vi "ReadFITS2SGL.vi"(8 "Error In":errorcluster, 11 "Path":path) -> (0 "error out":errorcluster, 1 "Tableau2DSGL":sgl[][][](array[numeric]), 2 "Tableau2DSGL":sgl[][](array[numeric]), 3 "Tableau_1D_SGL":sgl[](array[numeric]))   [LabVIEW 2020]
doc: "Relecture de fichier FITS. \nLes données sont relues au format SGL. Il y a un problème avec la lecture des données en U16. On les relit comme des entiers signés et j'ajoute la valeur 32768."
panel:
  out "Header":T1={"Naxis"=0, "Naxis1"=0, "Naxis2"=0, "Naxis3"=0, "DataType"=32, "Bscale"=0.0, "Bzero"=0.0} {"DataType" items=["U8"=8, "I16"=16, "I32"=32, "SGL (float)"=-32, "DBL"=-64]}
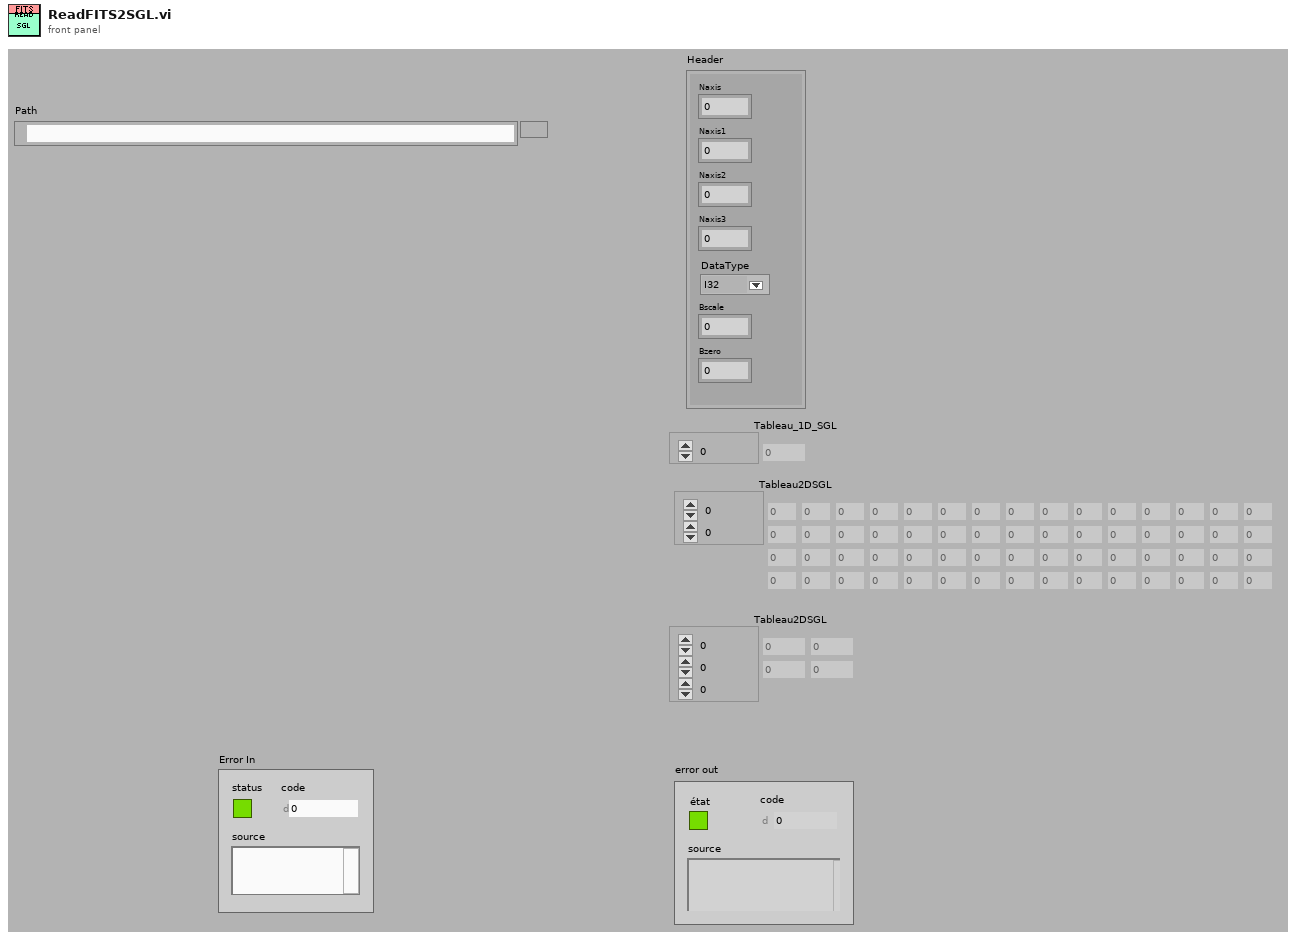
[diagram p1: front panel]
types:
  T1 = cluster{"Naxis":i32, "Naxis1":i32, "Naxis2":i32, "Naxis3":i32, "DataType":i32, "Bscale":dbl, "Bzero":dbl}
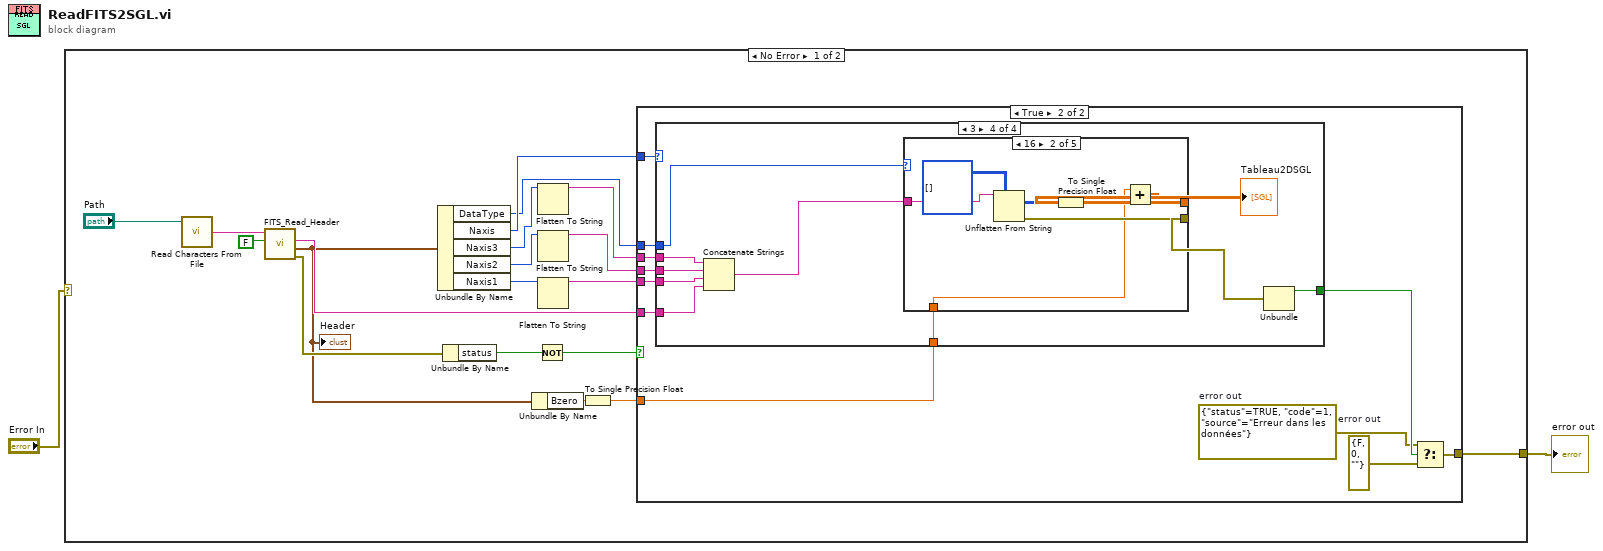
[diagram p0: block diagram]
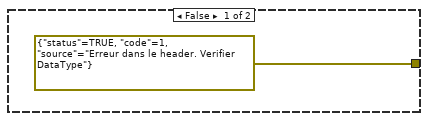
[diagram p2: hidden frame]
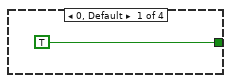
[diagram p3: hidden frame]
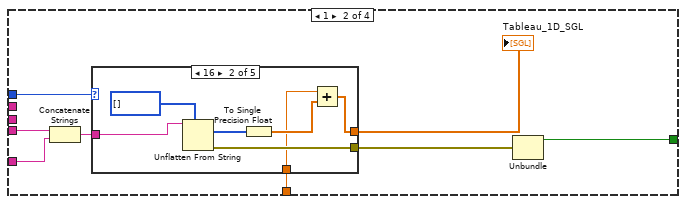
[diagram p4: hidden frame]
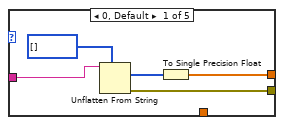
[diagram p5: hidden frame]
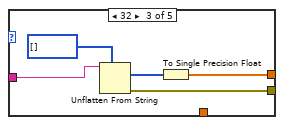
[diagram p6: hidden frame]
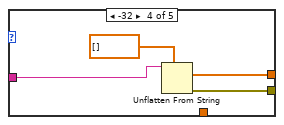
[diagram p7: hidden frame]
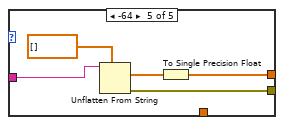
[diagram p8: hidden frame]
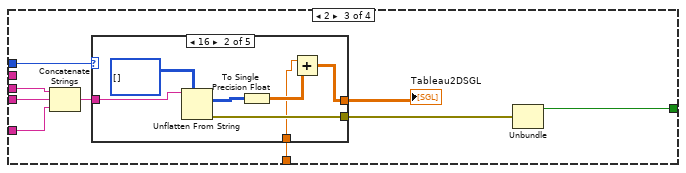
[diagram p9: hidden frame]
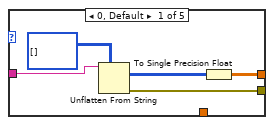
[diagram p10: hidden frame]
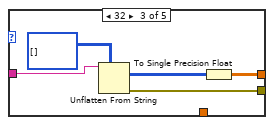
[diagram p11: hidden frame]
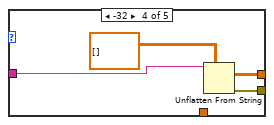
[diagram p12: hidden frame]
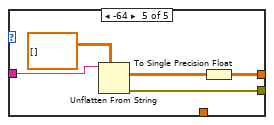
[diagram p13: hidden frame]
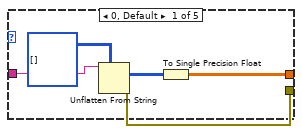
[diagram p14: hidden frame]
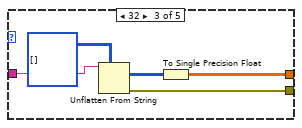
[diagram p15: hidden frame]
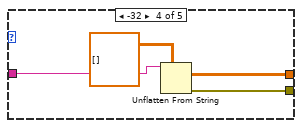
[diagram p16: hidden frame]
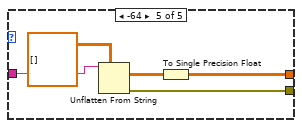
[diagram p17: hidden frame]
diagram:
  n1 = case shown="No Error" "Error In" {
    selector: "Error In" -> [_ w140]
    tunnel: [w6 w140] -> w2
    frame No Error {
      n2 = call <vilib>:"Read Characters From File.vi"("file path (dialog if empty)"="Path") -> ("character string"=w9:string)  [unwired: 5 in, 3 out]
      n3 = call "FITS_Read_Header.vi"("Load ?"=FALSE, "FITS in"=w9) -> ("error out"=w20:errorcluster, "Header"=w5:T1, "FITS data"=w15:string)  [unwired: 2 in, 1 out]
      "Header" <- w5
      n4 = Unbundle By Name(w5) -> ("DataType"=w7:i32, "Naxis"=w18:i32, "Naxis3"=w12:i32, "Naxis2"=w13:i32, "Naxis1"=w14:i32)
      n5 = Unbundle By Name(w20) -> ("status"=w19:bool)
      n6 = Unbundle By Name(w5) -> ("Bzero"=w4:dbl)
      n7 = Not(x=w19) -> (.not. x?=w10:bool)
      n8 = Flatten To String(anything=w12) -> (data string=w11:string)  [unwired: 3 in, 2 out]
      n9 = Flatten To String(anything=w13) -> (data string=w16:string)  [unwired: 3 in, 2 out]
      n10 = Flatten To String(anything=w14) -> (data string=w17:string)  [unwired: 3 in, 2 out]
      n11 = To Single Precision Float(number=w4) -> (single precision float=w3:sgl)
      n12 = case shown="True" w10 {
        tunnel: w17 -> [_ w32]
        tunnel: w18 -> [_ w33]
        tunnel: [errorcluster {"status"=TRUE, "code"=1, "source"="Erreur dans le header. Verifier DataType"} ("error out") w28] -> w6
        tunnel: w15 -> [_ w27]
        tunnel: w16 -> [_ w26]
        tunnel: w11 -> [_ w25]
        tunnel: w7 -> [_ w24]
        tunnel: w3 -> [_ w23]
        frame False {
        }
        frame True {
          w29 = errorcluster {"status"=TRUE, "code"=1, "source"="Erreur dans les données"}  # error out
          w30 = errorcluster {"status"=FALSE, "code"=0, "source"=""}  # error out
          n13 = case shown="3" w33 {
            tunnel: w32 -> [_ w41 w74 w111]
            tunnel: [TRUE ("err") w42 w77 w113] -> w31
            tunnel: w27 -> [_ w40 w75 w112]
            tunnel: w26 -> [_ _ w73 w110]
            tunnel: w25 -> [_ _ _ w109]
            tunnel: w24 -> [_ w37 w71 w105]
            tunnel: w23 -> [_ w35 w69 w104]
            frame 0, Default {
            }
            frame 1 {
              n14 = Concatenate Strings(w41, w40) -> (w39:string)
              n15 = case shown="16" w37 {
                tunnel: [w47 w54 w59 w63 w68] -> w38
                tunnel: w39 -> [w46 w53 w58 w62 w67]
                tunnel: [w44 w49 w55 w60 w64] -> w36
                tunnel: w35 -> [_ w48 _ _ _]
                frame 0, Default {
                  n16 = Unflatten From String(type=u8[] [] ("Tableau 3D SGL"), binary string=w46) -> (value=w43:u8[], error out=w47:errorcluster)  [unwired: 3 in, 1 out]
                  n17 = To Single Precision Float(number=w43) -> (single precision float=w44:sgl[])
                }
                frame 16 {
                  n18 = Unflatten From String(type=i16[] [] ("Tableau 3D SGL"), binary string=w53) -> (value=w51:i16[], error out=w54:errorcluster)  [unwired: 3 in, 1 out]
                  n19 = To Single Precision Float(number=w51) -> (single precision float=w50:sgl[])
                  n20 = Add(x=w48, y=w50) -> (x+y=w49:sgl[])
                }
                frame 32 {
                  n21 = Unflatten From String(type=i32[] [] ("Tableau 3D SGL"), binary string=w58) -> (value=w56:i32[], error out=w59:errorcluster)  [unwired: 3 in, 1 out]
                  n22 = To Single Precision Float(number=w56) -> (single precision float=w55:sgl[])
                }
                frame -32 {
                  n23 = Unflatten From String(type=sgl[] [] ("Tableau 3D SGL"), binary string=w62) -> (value=w60:sgl[], error out=w63:errorcluster)  [unwired: 3 in, 1 out]
                }
                frame -64 {
                  n24 = Unflatten From String(type=dbl[] [] ("Tableau 3D SGL"), binary string=w67) -> (value=w65:dbl[], error out=w68:errorcluster)  [unwired: 3 in, 1 out]
                  n25 = To Single Precision Float(number=w65) -> (single precision float=w64:sgl[])
                }
              }
              "Tableau_1D_SGL" <- w36
              n26 = Unbundle(w38) -> ("status"=w42:bool)  [unwired: 2 out]
            }
            frame 2 {
              n27 = Concatenate Strings(w73, w74, w75) -> (w72:string)
              n28 = case shown="16" w71 {
                tunnel: [w82 w89 w94 w98 w103] -> w76
                tunnel: w72 -> [w81 w88 w93 w97 w102]
                tunnel: [w79 w85 w90 w95 w99] -> w70
                tunnel: w69 -> [_ w83 _ _ _]
                frame 0, Default {
                  n29 = Unflatten From String(type=u8[][] [] ("Tableau 3D SGL"), binary string=w81) -> (value=w78:u8[][], error out=w82:errorcluster)  [unwired: 3 in, 1 out]
                  n30 = To Single Precision Float(number=w78) -> (single precision float=w79:sgl[][])
                }
                frame 16 {
                  n31 = Unflatten From String(type=i16[][] [] ("Tableau 3D SGL"), binary string=w88) -> (value=w86:i16[][], error out=w89:errorcluster)  [unwired: 3 in, 1 out]
                  n32 = To Single Precision Float(number=w86) -> (single precision float=w84:sgl[][])
                  n33 = Add(x=w83, y=w84) -> (x+y=w85:sgl[][])
                }
                frame 32 {
                  n34 = Unflatten From String(type=i32[][] [] ("Tableau 3D SGL"), binary string=w93) -> (value=w91:i32[][], error out=w94:errorcluster)  [unwired: 3 in, 1 out]
                  n35 = To Single Precision Float(number=w91) -> (single precision float=w90:sgl[][])
                }
                frame -32 {
                  n36 = Unflatten From String(type=sgl[][] [] ("Tableau 3D SGL"), binary string=w97) -> (value=w95:sgl[][], error out=w98:errorcluster)  [unwired: 3 in, 1 out]
                }
                frame -64 {
                  n37 = Unflatten From String(type=dbl[][] [] ("Tableau 3D SGL"), binary string=w102) -> (value=w100:dbl[][], error out=w103:errorcluster)  [unwired: 3 in, 1 out]
                  n38 = To Single Precision Float(number=w100) -> (single precision float=w99:sgl[][])
                }
              }
              "Tableau2DSGL" <- w70
              n39 = Unbundle(w76) -> ("status"=w77:bool)  [unwired: 2 out]
            }
            frame 3 {
              n40 = Concatenate Strings(w109, w110, w111, w112) -> (w107:string)
              n41 = case shown="16" w105 {
                tunnel: [w118 w125 w130 w134 w139] -> w106
                tunnel: w107 -> [w117 w124 w129 w133 w138]
                tunnel: [w114 w120 w126 w131 w135] -> w108
                tunnel: w104 -> [_ w119 _ _ _]
                frame 0, Default {
                  n42 = Unflatten From String(type=u8[][][] [] ("Tableau 3D SGL"), binary string=w117) -> (value=w115:u8[][][], error out=w118:errorcluster)  [unwired: 3 in, 1 out]
                  n43 = To Single Precision Float(number=w115) -> (single precision float=w114:sgl[][][])
                }
                frame 16 {
                  n44 = Unflatten From String(type=i16[][][] [] ("Tableau 3D SGL"), binary string=w124) -> (value=w122:i16[][][], error out=w125:errorcluster)  [unwired: 3 in, 1 out]
                  n45 = To Single Precision Float(number=w122) -> (single precision float=w121:sgl[][][])
                  n46 = Add(x=w119, y=w121) -> (x+y=w120:sgl[][][])
                }
                frame 32 {
                  n47 = Unflatten From String(type=i32[][][] [] ("Tableau 3D SGL"), binary string=w129) -> (value=w127:i32[][][], error out=w130:errorcluster)  [unwired: 3 in, 1 out]
                  n48 = To Single Precision Float(number=w127) -> (single precision float=w126:sgl[][][])
                }
                frame -32 {
                  n49 = Unflatten From String(type=sgl[][][] [] ("Tableau 3D SGL"), binary string=w133) -> (value=w131:sgl[][][], error out=w134:errorcluster)  [unwired: 3 in, 1 out]
                }
                frame -64 {
                  n50 = Unflatten From String(type=dbl[][][] [] ("Tableau 3D SGL"), binary string=w138) -> (value=w136:dbl[][][], error out=w139:errorcluster)  [unwired: 3 in, 1 out]
                  n51 = To Single Precision Float(number=w136) -> (single precision float=w135:sgl[][][])
                }
              }
              "Tableau2DSGL" <- w108
              n52 = Unbundle(w106) -> ("status"=w113:bool)  [unwired: 2 out]
            }
          }
          n53 = Select(t=w29, s=w31, f=w30) -> (s? t:f=w28:errorcluster)
        }
      }
    }
    frame Error {
    }
  }
  "error out" <- w2
